vi "API String - Remove Boolean Strings.vi"(8 "Error in":errorcluster caption="Error in (no error)", 10 "Custom False Boolean Strings":string[](array[string]), 11 "Custom True Boolean Strings":string[](array[string])) -> (0 "Error out":errorcluster, 2 "False Boolean Strings":string[](array[string]), 3 "True Boolean Strings":string[](array[string]))   [LabVIEW 2017, in "API String Arguments Support.lvlib"]
doc: "Removes custom boolean strings from the API String boolean parsing list and returns the updated list.\n\n\n> [!NOTE] <b>Default Strings for TRUE Value</b>\n>\n> Supports `1`, `Active`, `Enable`, `Non-null`, `On`, `T`, `True`, `valid`, `yes`.\n>\n> Case insensitive.\n\n\n> [!NOTE] <b>Default Strings for FALSE Value</b>\n>\n> Supports `0`, `Disable`, `F`, `False`, `Inactive`, `Invalid`, `No`, `Off`, `Void`, `null`.\n>\n> Case insensitive.\n\n\n-- <b>Controls</b> --\n- <b>Custom False Boolean Strings</b>: List of FALSE strings to remove.\n- <b>Custom True Boolean Strings</b>: List of TRUE strings to remove.\n\n-- <b>Indicators</b> --\n- <b>False Boolean Strings</b>: Updated list of FALSE strings.\n- <b>True Boolean Strings</b>: Updated list of TRUE strings."
uses:
  API String Arguments Support.lvlib
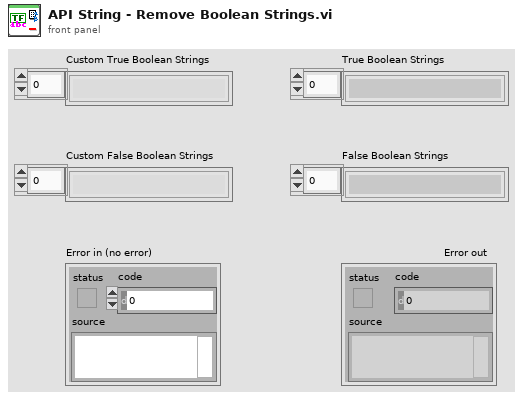
[diagram p1: front panel]
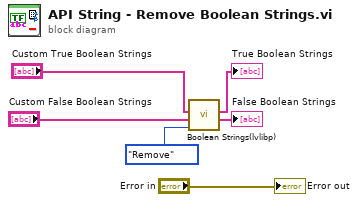
[diagram p0: block diagram]
diagram:
  n1 = call "Boolean Strings(lvlibp).vi"("Enum"=enum16{"List", "Add", "Remove"}."Remove", "Customer False Boolean Strings"="Custom False Boolean Strings", "Customer True Boolean Strings"="Custom True Boolean Strings") -> ("False Boolean Strings"=→"False Boolean Strings":string[], "True Boolean Strings"=→"True Boolean Strings":string[])  [unwired: 5 in, 2 out]
  "Error out" <- "Error in"
